vi "Detector Process File.vi"(8 "error in (no error)":errorcluster, 9 "Observation":T1={"Priority"=0, "ID"="", "Observer"="", "Obj Name"="", "Obj Type"="", "RA and DEC String"={"RA"="HH:MM:SS.nnn", "DEC"="DEG:arcmin:arcsec.nn"}, "Filters"=[], "Integration Time"=0.0, "Observation Status"=enum."Error", "Offsets"={"RA"=0.0, "DEC"=0.0, "ROT"=0.0}, "Images"=0, "Dither Options"={"Dither"=enum."None", "Dither Radius"=0.0, "Dither Points"=0, "Dither Phase"=0.0, "B Offset"={"RA"=0.0, "DEC"=0.0}}, "Comment 1"="", "Comment 2"=""}, 10 "Detector Config":T7={"Detector"=0, "Offsets"=[[0, 0, 0, 0, 0, 0, 0, 0, 0, 0, 0, 0, 0, 0, 0, 0, 0, 0, 0, 0, 0, 0, 0, 0, 0, 0, 0, 0, 0, 0, 0, 0]], "Detector Computer"={"Machine"="192.168.121.11", "Password"="rSL!nux23456", "FITS File Path"="", "Port"=44444, "Header Path"="", "Name"=""}, "FITS hdr template0"=path "", "FITS hdr template1"=path "", "FITS Data File Path"=path "", "FITS Detector Settings"={"Exp Time Short"=0.0, "# of Frames"=0.0, "Exp Time Long"=0.0, "# of Groups"=0.0, "Object Name"="", "Object"="", "Obs Type"="", "Image Type"="", "Observer"="", "Observer Affiliation"=""}, "Sim Folder"=path "", "Integration Mode"=enum."Ramp", "Integration Time"=0.0, "Frame Int Time"=0.0} {"Offsets" format="%04x"; "Detector" items=["0", "1", "2"]}, 11 "Image":T11) -> (0 "error out":errorcluster, 3 "FITS file":path)   [LabVIEW 2024]
uses:
  Detector Image typedef cluster.ctl
  RIMAS Detector Config.ctl
  RIMAS Detector Server Config.ctl
  RIMAS Observation Config.ctl
  Detector enum Detector Integration Mode.ctl
  typedefs/CC cluster Observation.ctl
  Observation Queue/CC enum Observation Status.ctl
  Telescope/CC cluster Telescope Offsets.ctl
  typedefs/CC cluster Observation Dither Options.ctl
  typedefs/CC enum Dither Selection.ctl
  typedefs/CC cluster RA and DEC.ctl
  d4ad78c3-49b1-47e4-a5d3-cc076b9db9ff.vi
  d0ebeae3-fb4d-4b72-85e7-31abb6c5fb53.vi
  8dbc6553-ea81-403b-9711-466f6854e3de.vi
  532e773a-19a8-4b9a-b404-3b26ad4e85e4.vi
  11e449f2-433d-42a2-a2be-b2367b0314ae.vi
  2a5e4c79-edeb-4c0d-9242-d248b7fccf42.vi
  59404dfe-7624-4c5d-9ba2-f9b135feb5fc.vi
  6fe851e7-a976-415e-b9db-a77fc37c1260.vi
  gfitsio/gfitsio-write-key-integer.vi
  gfitsio/gfitsio-write-key-string.vi
  gfitsio/gfitsio-write-key-double.vi
  gfitsio/gfitsio.lvlib
  PRIME Detector.lvclass
  Detector Class.lvclass
panel:
  out "Waveform Chart":cluster{u32, u32, u32, u32, u32, u32, u32}(graph)
  out "close":u32
  out "open":u32
  out "hdr":u32
  out "filters":u32
  out "hk":u32
  out "obs":u32
  out "obs stat":u32
  out "duration":u32
  # "sec"
  # "sec"
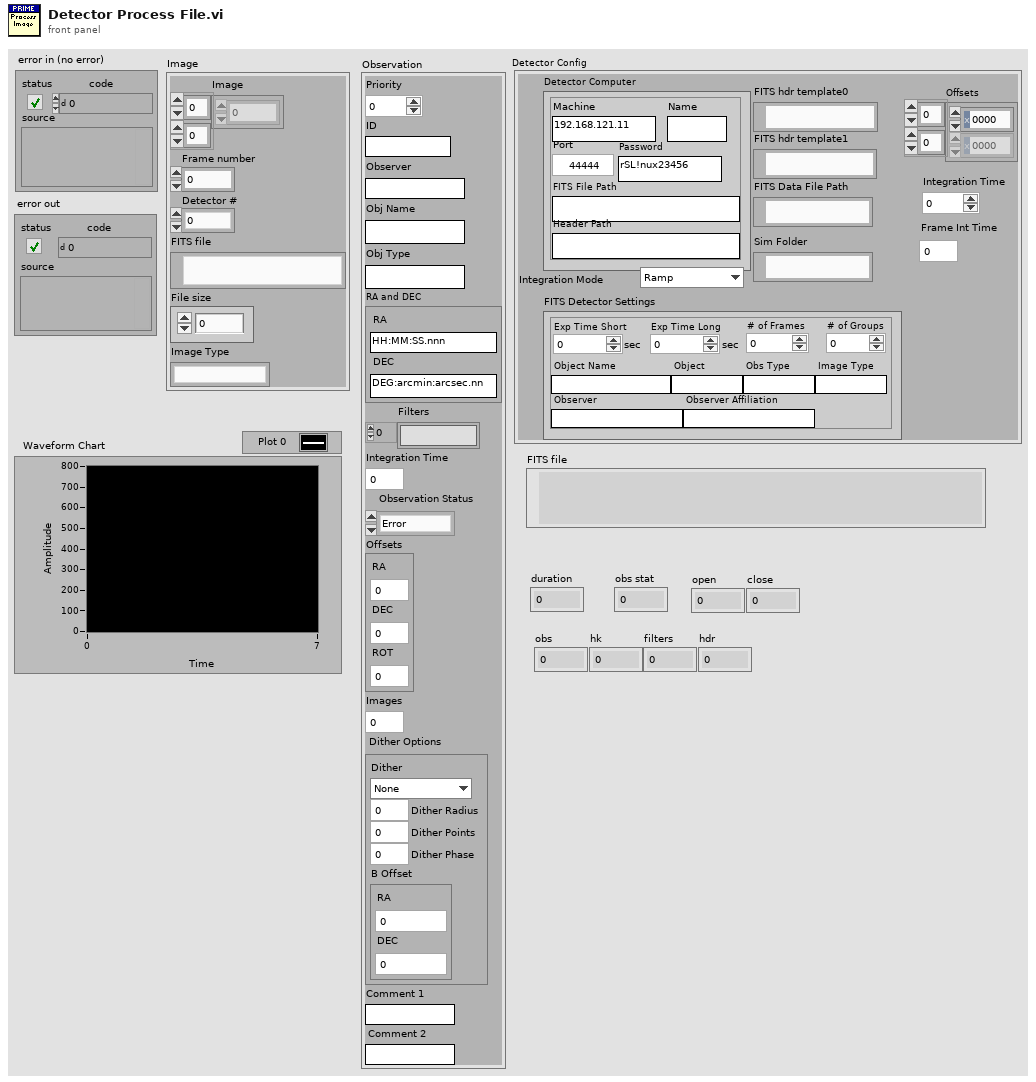
[diagram p1: front panel]
types:
  T1 = typedef "CC cluster Observation.ctl" = cluster{"Priority":i32, "ID":string, "Observer":string, "Obj Name":string, "Obj Type":string, "RA and DEC String":cluster{"RA":string, "DEC":string}, "Filters":string[], "Integration Time":dbl, "Observation Status":T2, "Offsets":T3, "Images":i32, "Dither Options":T4, "Comment 1":string, "Comment 2":string}
  T2 = typedef "CC enum Observation Status.ctl" = enum16{"Ready", "Running", "Done", "Error"}
  T3 = typedef "CC cluster Telescope Offsets.ctl" = cluster{"RA":dbl, "DEC":dbl, "ROT":dbl}
  T4 = typedef "CC cluster Observation Dither Options.ctl" = cluster{"Dither":T5, "Dither Radius":dbl, "Dither Points":i32, "Dither Phase":dbl, "B Offset":T6}
  T5 = typedef "CC enum Dither Selection.ctl" = enum16{"None", "Circle", "Random", "ABBA"}
  T6 = typedef "CC cluster RA and DEC.ctl" = cluster{"RA":dbl, "DEC":dbl}
  T7 = typedef "RIMAS Detector Config.ctl" = cluster{"Detector":u16, "Offsets":u16[][], "Detector Computer":T8, "FITS hdr template0":path, "FITS hdr template1":path, "FITS Data File Path":path, "FITS Detector Settings":T9, "Sim Folder":path, "Integration Mode":T10, "Integration Time":dbl, "Frame Int Time":dbl}
  T8 = typedef "RIMAS Detector Server Config.ctl" = cluster{"Machine":string, "Password":string, "FITS File Path":string, "Port":u16, "Header Path":string, "Name":string}
  T9 = typedef "RIMAS Observation Config.ctl" = cluster{"Exp Time Short":dbl, "# of Frames":dbl, "Exp Time Long":dbl, "# of Groups":dbl, "Object Name":string, "Object":string, "Obs Type":string, "Image Type":string, "Observer":string, "Observer Affiliation":string}
  T10 = typedef "Detector enum Detector Integration Mode.ctl" = enum16{"Ramp", "CDS", "FOWLER2", "FOWLER4", "FOWLER8", "FOWLER16", "Raw"}
  T11 = typedef "Detector Class.lvclass/Detector Image typedef cluster.ctl" = cluster{"Image":sgl[][], "Frame number":i32, "Detector #":u16, "FITS file":path, "File size":i64, "Image Type":string}
  T12 = typedef "FITS cluster Header Row.ctl" = cluster{"Field Name":string, "Type":T13, "Value":string, "Comment":string, "Units":string}
  T13 = typedef "FITS enum Data Type.ctl" = enum16{"String", "Integer", "Float"}
  T14 = typedef "gfitsio.lvlib/gfitsio-refnum.ctl" = u64
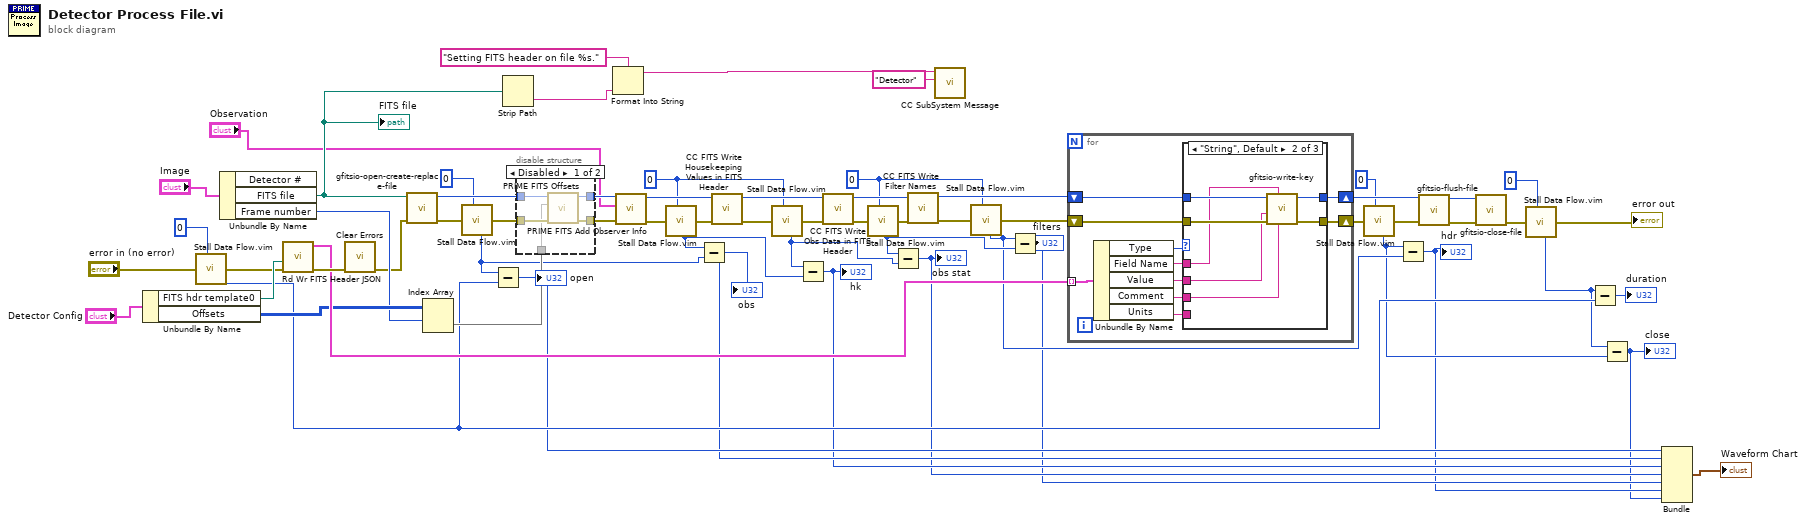
[diagram p0: block diagram]
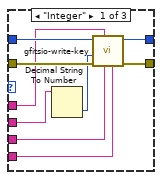
[diagram p3: hidden frame]
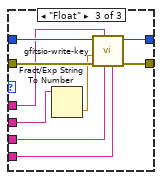
[diagram p4: hidden frame]
diagram:
  w21 = u32 0 ("milliseconds to wait")
  w20 = u32 0 ("milliseconds to wait")
  n1 = Unbundle By Name("Detector Config") -> ("FITS hdr template0"=w37:path, "Offsets"=w41:u16[][])
  n2 = call "Stall Data Flow.vim"("value in"="error in (no error)", "milliseconds to wait"=u32 0) -> ("millisecond timer value"=w16:u32, "value out"=w31:errorcluster)
  n3 = Unbundle By Name("Image") -> ("FITS file"=w50:path, "Frame number"=w40:i32)  [unwired: 1 out]
  "FITS file" <- w50
  n4 = call "Rd Wr FITS Header JSON.vi"("error in (no error)"=w31, "FITS Template"=w37) -> ("error out"=w44:errorcluster, "FITS Hdr Rows"=w42:T12[])  [unwired: 8 in]
  n5 = call <vilib>:"Clear Errors.vi"("error in (no error)"=w44) -> ("error out"=w36:errorcluster)  [unwired: 5 in, 1 out]
  n6 = call "gfitsio-open-create-replace-file.vi"("error in (no error)"=w36, "file path (dialog if empty)"=w50) -> ("error out"=w64:errorcluster, "gfits refnum"=w63:T14)  [unwired: 7 in, 1 out]
  n7 = Index Array(array=w41, index (row)=w40) -> (element=w58:u16[])  [unwired: 1 in]
  n8 = call "Stall Data Flow.vim"("value in"=w64, "milliseconds to wait"=u32 0) -> ("millisecond timer value"=w15:u32, "value out"=w18:errorcluster)
  n9 = Subtract(x=w15, y=w16) -> (x-y=w8:u32)
  "open" <- w8
  n10 = Strip Path(path=w50) -> (name=w49:string)  [unwired: 1 out]
  n11 = disable-structure shown="Disabled" {
    disable-tunnel: w18 -> [w69 w70]
    disable-tunnel: w63 -> [w68 w71]
    disable-tunnel: [w67 w71] -> w62
    disable-tunnel: [w66 w70] -> w61
    disable-tunnel: w58 -> [w65 _]
    frame Disabled {
      n12 = call "PRIME FITS Offsets.vi"("error in (no error)"=w69, "Offsets"=w65, "gfits refnum"=w68) -> ("error out"=w66:errorcluster, "gfits refnum out"=w67:T14)  [unwired: 7 in]
    }
    frame Enabled {
    }
  }
  n13 = Format Into String(format string="Setting FITS header on file %s.", w49) -> (resulting string=w47:string)  [unwired: 2 in, 1 out]
  n14 = call "PRIME FITS Add Observer Info.vi"("Error In"=w61, "Observation"="Observation", "gfits refnum"=w62) -> ("Error Out"=w55:errorcluster, "dup gfits refnum"=w54:T14)  [unwired: 7 in]
  n15 = call "Stall Data Flow.vim"("value in"=w55, "milliseconds to wait"=w21) -> ("millisecond timer value"=w14:u32, "value out"=w25:errorcluster)
  n16 = Subtract(x=w14, y=w15) -> (x-y=w7:u32)
  "obs" <- w7
  n17 = call "CC FITS Write Housekeeping Values in FITS Header.vi"("error in (no error)"=w25, "gfits refnum"=w54) -> ("error out"=w35:errorcluster, "dup gfits refnum"=w34:T14)  [unwired: 8 in]
  n18 = call "Stall Data Flow.vim"("value in"=w35, "milliseconds to wait"=w21) -> ("millisecond timer value"=w13:u32, "value out"=w24:errorcluster)
  n19 = Subtract(x=w13, y=w14) -> (x-y=w6:u32)
  "hk" <- w6
  n20 = call "CC FITS Write Obs Data in FITS Header.vi"("error in (no error)"=w24, "gfits refnum"=w34) -> ("error out"=w32:errorcluster, "dup gfits refnum"=w33:T14)  [unwired: 8 in]
  n21 = call "Stall Data Flow.vim"("value in"=w32, "milliseconds to wait"=w20) -> ("millisecond timer value"=w12:u32, "value out"=w26:errorcluster)
  n22 = Subtract(x=w12, y=w13) -> (x-y=w5:u32)
  "obs stat" <- w5
  n23 = call "CC FITS Write Filter Names.vi"("error in (no error)"=w26, "gfits refnum"=w33) -> ("error out"=w53:errorcluster, "dup gfits refnum"=w52:T14)  [unwired: 8 in]
  n24 = call "CC SubSystem Message.vi"("Subsystem"="Detector", "Message"=w47) -> ()  [unwired: 9 in, 1 out]
  n25 = call "Stall Data Flow.vim"("value in"=w53, "milliseconds to wait"=w20) -> ("millisecond timer value"=w11:u32, "value out"=w23:errorcluster)
  n26 = Subtract(x=w11, y=w12) -> (x-y=w4:u32)
  "filters" <- w4
  n27 = for {
    shift-right: [w78] -> w57
    shift-left: w52 -> [w80]
    shift-right: [w77] -> w56
    shift-left: w23 -> [w79]
    tunnel: w42 -> [w81] mode=indexing
    n28 = Unbundle By Name(w81) -> ("Type"=w76:T13, "Field Name"=w75:string, "Value"=w73:string, "Comment"=w74:string, "Units"=w72:string)
    n29 = case shown="\"String\", Default" w76 {
      tunnel: w80 -> [w90 w97 w106]
      tunnel: w79 -> [w89 w96 w105]
      tunnel: [w88 w95 w104] -> w78
      tunnel: [w87 w94 w103] -> w77
      tunnel: w75 -> [w86 w93 w102]
      tunnel: w74 -> [w85 w92 w101]
      tunnel: w73 -> [w84 w91 w100]
      tunnel: w72 -> [w82 _ w98]
      frame "Integer" {
        n30 = Decimal String To Number(string=w84) -> (number=w83:i32)  [unwired: 2 in, 1 out]
        n31 = call-poly "gfitsio-write-key.vi"("units"=w82, "comment"=w85, "keyname"=w86, "error in (no error)"=w89, "value"=w83, "gfits refnum"=w90) -> ("error out"=w87:errorcluster, "dup gfits refnum"=w88:T14)  [unwired: 4 in]
      }
      frame "String", Default {
        n32 = call-poly "gfitsio-write-key.vi"("comment"=w92, "keyname"=w93, "error in (no error)"=w96, "value"=w91, "gfits refnum"=w97) -> ("error out"=w94:errorcluster, "dup gfits refnum"=w95:T14)  [unwired: 5 in]
      }
      frame "Float" {
        n33 = Fract/Exp String To Number(string=w100) -> (number=w99:dbl)  [unwired: 3 in, 1 out]
        n34 = call-poly "gfitsio-write-key.vi"("units"=w98, "comment"=w101, "keyname"=w102, "error in (no error)"=w105, "value"=w99, "gfits refnum"=w106) -> ("error out"=w103:errorcluster, "dup gfits refnum"=w104:T14)  [unwired: 4 in]
      }
    }
  }
  n35 = call "Stall Data Flow.vim"("value in"=w56, "milliseconds to wait"=u32 0) -> ("millisecond timer value"=w9:u32, "value out"=w22:errorcluster)
  n36 = Subtract(x=w9, y=w11) -> (x-y=w3:u32)
  "hdr" <- w3
  n37 = call "gfitsio-flush-file.vi"("error in (no error)"=w22, "gfits refnum"=w57) -> ("error out"=w60:errorcluster, "dup gfits refnum"=w59:T14)  [unwired: 8 in]
  n38 = call "gfitsio-close-file.vi"("error in (no error)"=w60, "gfits refnum"=w59) -> ("error out"=w38:errorcluster)  [unwired: 8 in, 1 out]
  n39 = call "Stall Data Flow.vim"("value in"=w38, "milliseconds to wait"=u32 0) -> ("millisecond timer value"=w10:u32, "value out"=→"error out":errorcluster)
  n40 = Subtract(x=w10, y=w16) -> (x-y=→"duration":u32)
  n41 = Subtract(x=w10, y=w9) -> (x-y=w2:u32)
  "close" <- w2
  n42 = Bundle(w8, w7, w6, w5, w4, w3, w2) -> (→"Waveform Chart":cluster{u32, u32, u32, u32, u32, u32, u32})  [unwired: 1 in]
